vi "Kikusui PLZ-Configure Protection.vi"(5 "Enable UVP":bool, 7 "Enable Trip":bool, 8 "error in":errorcluster, 9 "Protection Limit (0)":dbl, 10 "Protection Type (0:OCP)":u16(ring) items=["Over Current Protection (OCP)", "Over Power Protection (OPP)", "Under Voltage Protection (UVP)"], 11 "Kikusui PLZ Setting In":T1={"VISA Resource Name"="", "Baud Rate"=19200, "Stop Bits"=20, "Wait For Read(ms)"=0} {"Stop Bits" items=["1.0"=10, "2.0"=20]; "Baud Rate" items=["2400"=2400, "4800"=4800, "9600"=9600, "19200"=19200]}) -> (0 "error out":errorcluster, 3 "Kikusui PLZ Setting Out":T1={"VISA Resource Name"="", "Baud Rate"=19200, "Stop Bits"=20, "Wait For Read(ms)"=0} {"Stop Bits" items=["1.0"=10, "2.0"=20]; "Baud Rate" items=["2400"=2400, "4800"=4800, "9600"=9600, "19200"=19200]})   [LabVIEW 2018]
doc: "Configures current, power or voltage protection. Whenever the current, power or voltage reaches the limit specified, it will either limit or turn off the load."
uses:
  Data Def/Kikusui PLZ-Setting.ctl
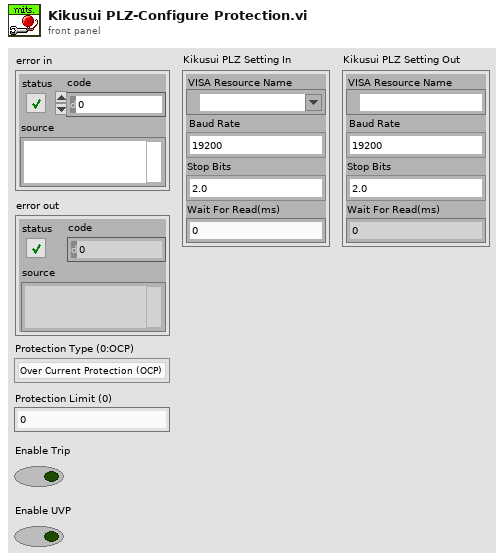
[diagram p1: front panel]
types:
  T1 = typedef "Kikusui PLZ-Setting.ctl" = cluster{"VISA Resource Name":refnum<visa-resource-name>, "Baud Rate":u32, "Stop Bits":u16, "Wait For Read(ms)":u32}
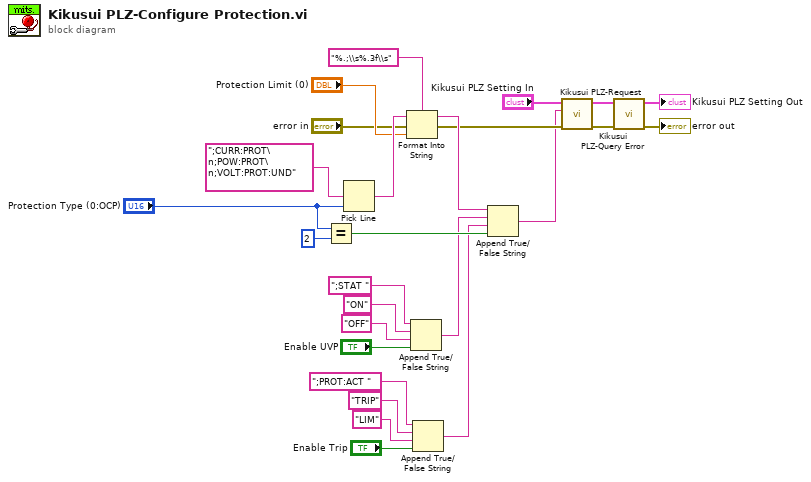
[diagram p0: block diagram]
diagram:
  n1 = Equal?(x="Protection Type (0:OCP)", y=u16 2) -> (x = y?=w18:bool)
  n2 = Pick Line(multi-line string=";CURR:PROT\n;POW:PROT\n;VOLT:PROT:UND", line index="Protection Type (0:OCP)") -> (output string=w24:string)  [unwired: 1 in]
  n3 = Format Into String(format string="%.;\\s%.3f\\s", initial string=w24, error in="error in", "Protection Limit (0)") -> (resulting string=w14:string, error out=w4:errorcluster)
  n4 = Append True/False String(1:"Enable UVP", 2:"OFF" ("false string"), 3:"ON" ("true string"), 4:";STAT " ("string (\"\")")) -> (0:w16:string)
  n5 = Append True/False String(1:"Enable Trip", 2:"LIM" ("false string"), 3:"TRIP" ("true string"), 4:";PROT:ACT " ("false string")) -> (0:w15:string)
  n6 = Append True/False String(1:w18, 2:w15, 3:w16, 4:w14) -> (0:w3:string)
  n7 = call "Kikusui PLZ-Request.vi"("error in"=w4, "Command"=w3, "Kikusui PLZ Setting In"="Kikusui PLZ Setting In") -> ("error out"=w6:errorcluster, "Kikusui PLZ Setting Out"=w5:T1)  [unwired: 6 in, 1 out]
  n8 = call "Kikusui PLZ-Query Error.vi"("error in"=w6, "Kikusui PLZ Setting In"=w5) -> ("error out"=→"error out":errorcluster, "Kikusui PLZ Setting Out"=→"Kikusui PLZ Setting Out":T1)  [unwired: 8 in]
